vi "PostSubDataSal.vi"(7 "newValue (T)":bool=TRUE, 8 "error in (no error)":errorcluster, 9 "value":variant, 10 "subDataSV":T1, 11 "MiddlewareSALThisComponent in":refnum<class "MiddlewareSALThisComponent.lvclass">) -> (0 "error out":errorcluster, 3 "MiddlewareSALThisComponent out":refnum<class "MiddlewareSALThisComponent.lvclass">)   [LabVIEW 2016, in "MiddlewareSALThisComponent.lvclass"]
uses:
  MiddlewareSALThisComponent.lvclass
  Typedefs/SubDataSignal.ctl
  ts_sallv_sedspectrometer/DataTypes/command_Disable.ctl
  ts_sallv_sedspectrometer/DataTypes/command_Enable.ctl
  ts_sallv_sedspectrometer/DataTypes/command_ExitControl.ctl
  ts_sallv_sedspectrometer/DataTypes/command_StandBy.ctl
  ts_sallv_sedspectrometer/DataTypes/command_Start.ctl
  ts_sallv_sedspectrometer/SALLV_calibrationSpectrometer.lvlib
  ProgrammaticInitialization/ProgrammaticInitialization.lvclass
  Typedefs/EXATypedefs.lvlib
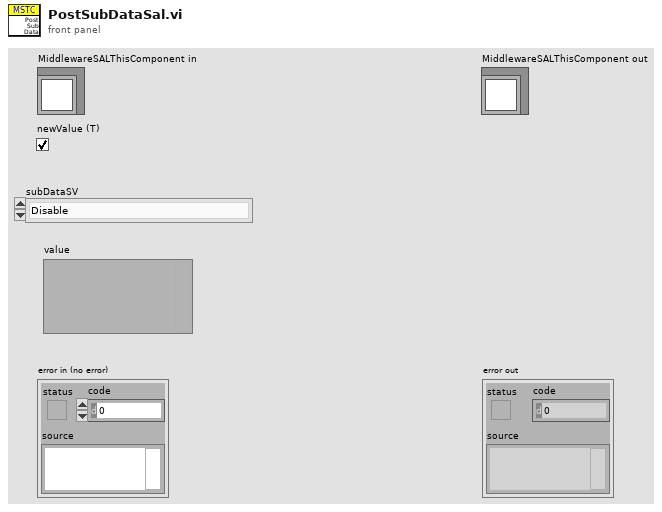
[diagram p1: front panel]
types:
  T1 = typedef "EXATypedefs.lvlib/SubDataSignal.ctl" = enum16{"Disable", "Enable", "Exit", "GoToStandby", "HeartbeatIn", "Start"}
  T2 = typedef "SALLV_calibrationSpectrometer.lvlib/command_Disable.ctl" = cluster{"disable":bool}
  T3 = typedef "SALLV_calibrationSpectrometer.lvlib/command_Enable.ctl" = cluster{"enable":bool}
  T4 = typedef "SALLV_calibrationSpectrometer.lvlib/command_ExitControl.ctl" = cluster{"exitControl":bool}
  T5 = typedef "SALLV_calibrationSpectrometer.lvlib/command_StandBy.ctl" = cluster{"standBy":bool}
  T6 = typedef "SALLV_calibrationSpectrometer.lvlib/command_Start.ctl" = cluster{"settingsToApply":string}
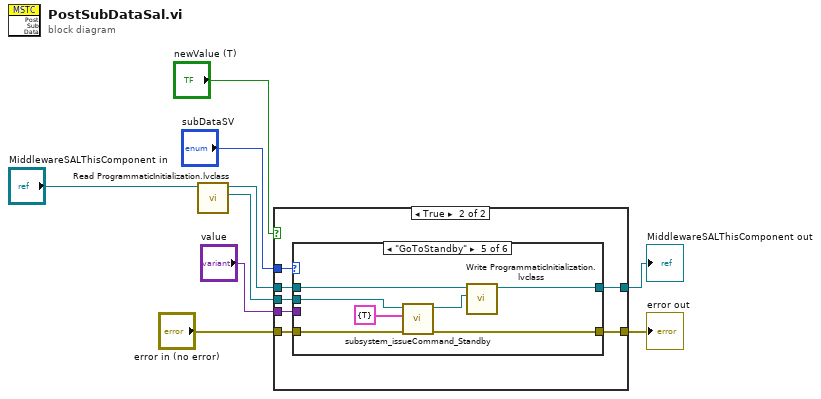
[diagram p0: block diagram]
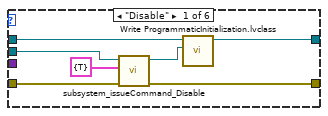
[diagram p3: hidden frame]
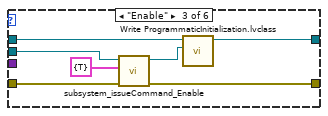
[diagram p5: hidden frame]
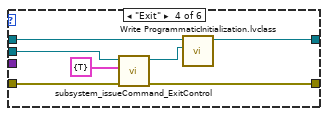
[diagram p6: hidden frame]
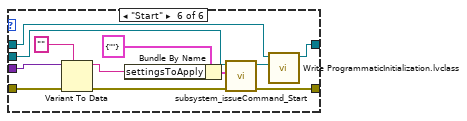
[diagram p7: hidden frame]
diagram:
  n1 = call-dynamic "Read ProgrammaticInitialization.lvclass.vi"("MiddlewareSALThisComponent in"="MiddlewareSALThisComponent in") -> ("ProgrammaticInitialization.lvclass"=w2:refnum<class "ProgrammaticInitialization.lvclass">, "MiddlewareSALThisComponent out"=w1:refnum<class "MiddlewareSALThisComponent.lvclass">)  [unwired: 8 in, 1 out]
  n2 = case shown="True" "newValue (T)" {
    tunnel: "subDataSV" -> [_ w18]
    tunnel: "error in (no error)" -> [w11 w17]
    tunnel: [w11 w16] -> w7
    tunnel: [w10 w15] -> w6
    tunnel: "value" -> [_ w14]
    tunnel: w2 -> [_ w13]
    tunnel: w1 -> [w10 w12]
    frame False {
    }
    frame True {
      n3 = case shown="\"GoToStandby\"" w18 {
        tunnel: w17 -> [w24 w27 w33 w40 w47 w58]
        tunnel: [w25 w27 w34 w41 w48 w52] -> w16
        tunnel: [w19 w26 w30 w37 w44 w49] -> w15
        tunnel: w14 -> [_ _ _ _ _ w59]
        tunnel: w13 -> [w22 _ w31 w38 w45 w55]
        tunnel: w12 -> [w21 w26 w28 w36 w43 w51]
        frame "Disable" {
          n4 = call "subsystem_issueCommand_Disable.vi"("error in (no error)"=w24, "command_Disable"=T2 {"disable"=TRUE} ("command_disable_Ctl"), "ProgrammaticInitialization in"=w22) -> ("error out"=w25:errorcluster, "ProgrammaticInitialization out"=w20:refnum<class "ProgrammaticInitialization.lvclass">)  [unwired: 7 in]
          n5 = call-dynamic "Write ProgrammaticInitialization.lvclass.vi"("ProgrammaticInitialization.lvclass"=w20, "MiddlewareSALThisComponent in"=w21) -> ("MiddlewareSALThisComponent out"=w19:refnum<class "MiddlewareSALThisComponent.lvclass">)  [unwired: 8 in, 1 out]
        }
        frame Default {
        }
        frame "Enable" {
          n6 = call "subsystem_issueCommand_Enable.vi"("error in (no error)"=w33, "command_Enable"=T3 {"enable"=TRUE} ("command_enable_Ctl"), "ProgrammaticInitialization in"=w31) -> ("error out"=w34:errorcluster, "ProgrammaticInitialization out"=w29:refnum<class "ProgrammaticInitialization.lvclass">)  [unwired: 7 in]
          n7 = call-dynamic "Write ProgrammaticInitialization.lvclass.vi"("ProgrammaticInitialization.lvclass"=w29, "MiddlewareSALThisComponent in"=w28) -> ("MiddlewareSALThisComponent out"=w30:refnum<class "MiddlewareSALThisComponent.lvclass">)  [unwired: 8 in, 1 out]
        }
        frame "Exit" {
          n8 = call "subsystem_issueCommand_ExitControl.vi"("error in (no error)"=w40, "command_ExitControl"=T4 {"exitControl"=TRUE} ("command_exitControl_Ctl"), "ProgrammaticInitialization in"=w38) -> ("error out"=w41:errorcluster, "ProgrammaticInitialization out"=w35:refnum<class "ProgrammaticInitialization.lvclass">)  [unwired: 7 in]
          n9 = call-dynamic "Write ProgrammaticInitialization.lvclass.vi"("ProgrammaticInitialization.lvclass"=w35, "MiddlewareSALThisComponent in"=w36) -> ("MiddlewareSALThisComponent out"=w37:refnum<class "MiddlewareSALThisComponent.lvclass">)  [unwired: 8 in, 1 out]
        }
        frame "GoToStandby" {
          n10 = call "subsystem_issueCommand_Standby.vi"("error in (no error)"=w47, "command_Standby"=T5 {"standBy"=TRUE} ("command_standby_Ctl"), "ProgrammaticInitialization in"=w45) -> ("error out"=w48:errorcluster, "ProgrammaticInitialization out"=w42:refnum<class "ProgrammaticInitialization.lvclass">)  [unwired: 7 in]
          n11 = call-dynamic "Write ProgrammaticInitialization.lvclass.vi"("ProgrammaticInitialization.lvclass"=w42, "MiddlewareSALThisComponent in"=w43) -> ("MiddlewareSALThisComponent out"=w44:refnum<class "MiddlewareSALThisComponent.lvclass">)  [unwired: 8 in, 1 out]
        }
        frame "Start" {
          n12 = Variant To Data(error in=w58, type="" ("data"), Variant=w59) -> (data=w56:string, error out=w53:errorcluster)
          n13 = Bundle By Name(cluster=T6 {"settingsToApply"=""} ("command_start_Ctl"), "settingsToApply"=w56) -> (w54:T6)
          n14 = call "subsystem_issueCommand_Start.vi"("error in (no error)"=w53, "command_Start"=w54, "ProgrammaticInitialization in"=w55) -> ("error out"=w52:errorcluster, "ProgrammaticInitialization out"=w50:refnum<class "ProgrammaticInitialization.lvclass">)  [unwired: 7 in]
          n15 = call-dynamic "Write ProgrammaticInitialization.lvclass.vi"("ProgrammaticInitialization.lvclass"=w50, "MiddlewareSALThisComponent in"=w51) -> ("MiddlewareSALThisComponent out"=w49:refnum<class "MiddlewareSALThisComponent.lvclass">)  [unwired: 8 in, 1 out]
        }
      }
    }
  }
  "error out" <- w7
  "MiddlewareSALThisComponent out" <- w6
